vi "q2 bcg control.vi"() -> ()   [LabVIEW 2018]
uses:
  <vilib>/vision/NI_Vision_Development_Module.lvlib
panel:
  in  "BCG Values":T1={"Brightness"=128.0, "Contrast"=45.0, "Gamma"=1.0} {"Brightness" min=0 max=255 step=1 format="%.2f"; "Contrast" min=1 max=89 step=1 format="%.2f"; "Gamma" min=0.1 max=10 step=0.01 format="%.2f"}
  out "Image 2":T2(plugin-control)
  in  "Interval Range":cluster{"Minimum":sgl, "Maximum":sgl} {"Maximum" format="%.2f"; "Minimum" format="%.2f"}
  out "Histogram Report":T3 {"Standard  Variation" format="%.2f"; "Mean Value" format="%.2f"; "Interval Width" format="%.2f"; "Starting Value" format="%.2f"; "Maximal Value" format="%.2f"; "Minimal Value" format="%.2f"}
  out "Waveform Graph":T4(graph)
  in  "Use File Path Image Type":bool=TRUE
  out "Image":T2(plugin-control)
  in  "File Path":path
  in  "Image Type":T5 items=["Grayscale (U8)", "Grayscale (I16)", "Grayscale (SGL)", "Complex (CSG)", "RGB (U32)", "HSL (U32)", "RGB (U64)", "Grayscale (U16)"]
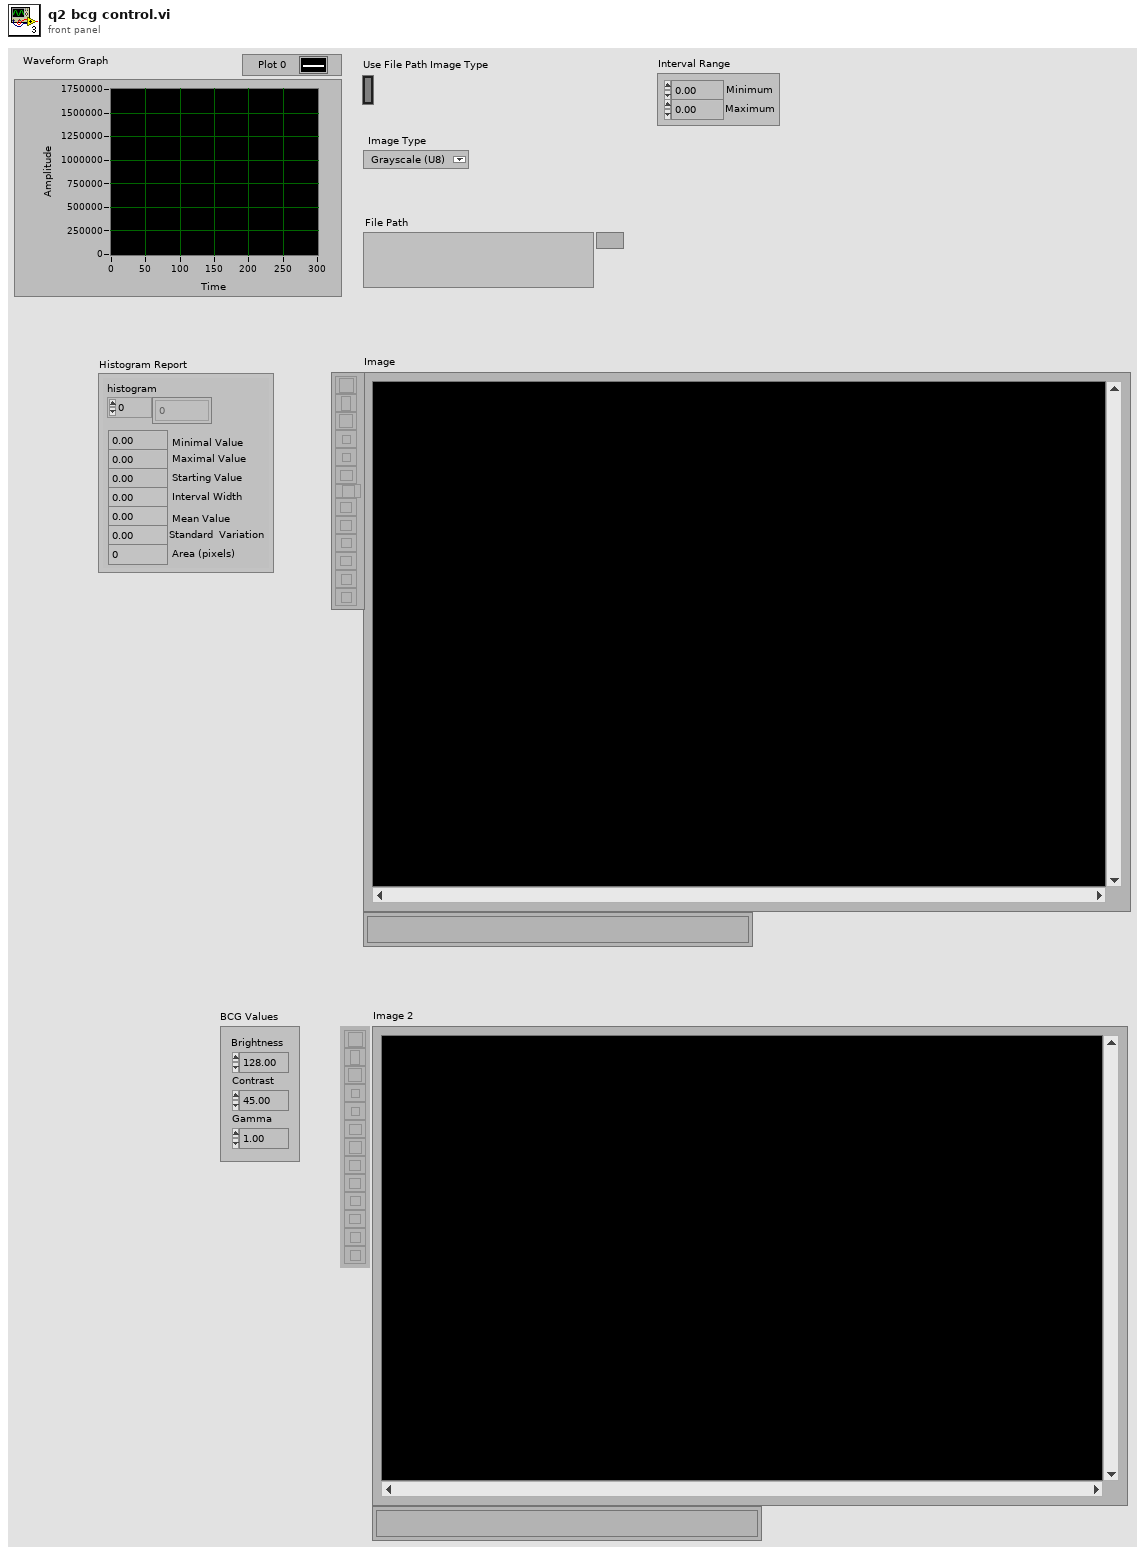
[diagram p1: front panel]
types:
  T1 = cluster{"Brightness":sgl, "Contrast":sgl, "Gamma":sgl}
  T2 = typedef "IMAQ Image.ctl" = refnum<image>
  T3 = cluster{"histogram":u32[], "Minimal Value":sgl, "Maximal Value":sgl, "Starting Value":sgl, "Interval Width":sgl, "Mean Value":sgl, "Standard  Variation":sgl, "Area (pixels)":i32}
  T4 = cluster{"Starting Value":sgl, "Incremental Value":sgl, "Histogram":u32[]}
  T5 = typedef "Image Type" = u32
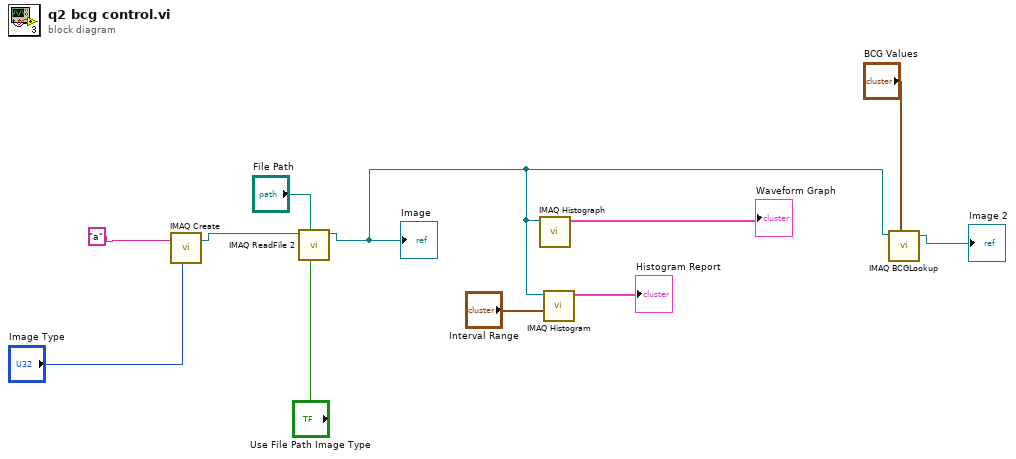
[diagram p0: block diagram]
diagram:
  n1 = call "IMAQ Create"("Image Name"="a", "Image Type"="Image Type") -> ("New Image"=w9:T2)  [unwired: 3 in, 1 out]
  n2 = call "IMAQ ReadFile 2"("Use File Path Image Type"="Use File Path Image Type", "File Path"="File Path", "Image"=w9) -> ("Image Out"=w3:T2)  [unwired: 4 in, 4 out]
  "Image" <- w3
  n3 = call "IMAQ Histograph"("Image"=w3) -> ("Histogram Graph"=→"Waveform Graph":T4)  [unwired: 7 in, 3 out]
  n4 = call "IMAQ Histogram"("Interval Range"="Interval Range", "Image"=w3) -> ("Histogram Report"=→"Histogram Report":T3)  [unwired: 8 in, 1 out]
  n5 = call "IMAQ BCGLookup"("Image Src"=w3, "BCG Values"="BCG Values") -> ("Image Dst Out"=→"Image 2":T2)  [unwired: 5 in, 1 out]
